vi "Find Refs.vi"(7 "Actor in":refnum<class "Actor.lvclass">) -> (2 "Refs":T1)   [LabVIEW 2020, in "_Template.lvlib" / "Templates.lvlib" / "TEMPLATE jettl Actor.lvlib" / "TEMPLATE Actor.lvlib" / "TEMPLATE Refs.lvlib"]
uses:
  TEMPLATE Refs.lvlib
  jettl/jettl/Actor/Actor.lvclass
  Refs.ctl
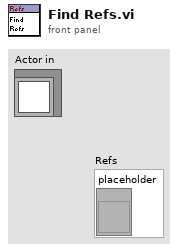
[diagram p1: front panel]
types:
  T1 = typedef "_Template.lvlib/Templates.lvlib/TEMPLATE jettl Actor.lvlib/TEMPLATE Actor.lvlib/TEMPLATE Refs.lvlib/Refs.ctl" = cluster{"placeholder":refnum<vi>}
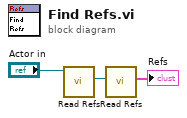
[diagram p0: block diagram]
diagram:
  n1 = call-dynamic "Read Refs.vi"("Actor in"="Actor in") -> ("Refs"=w3:refnum<class "Refs.lvclass">)  [unwired: 10 in]
  n2 = call "Read Refs.vi"("Refs"=w3) -> ("Refs"=→"Refs":T1)  [unwired: 10 in]
